vi "RunScript.vi"(6 "String Reference (Severity)":refnum<vi>, 7 "ScriptFileNames":path[](array[path]), 8 "Error In":errorcluster, 10 "File Path to Python Script":path, 11 "Python or INIScript?":T1=enum."Python") -> (0 "Error Out":errorcluster, 1 "Valid File Path":bool, 2 "File Path Control Out":path, 3 "Python Script Window":bool, 4 "INI Script Name Out":string)   [LabVIEW 2018]
doc: "This VI allows the which Script (Python or INI file) to run and/or whether to enable automatic error handling and leave the python script command window open to aid in debuging."
uses:
  TypeDefs/PythonOrINIScript.ctl
  NistPluggableModules/TestClass/Test.lvclass
panel:
  in  "INI Script Name":u16(ring) items=["*AbortScript", "*Start", "*Stop", "*AutoTimeout", "*Script", "*T", "*TT0", "*TT1"]
  in  "Cancel Button":bool
  in  "Auto In":bool
  in  "Done Button":bool
  in  "PSW In":bool
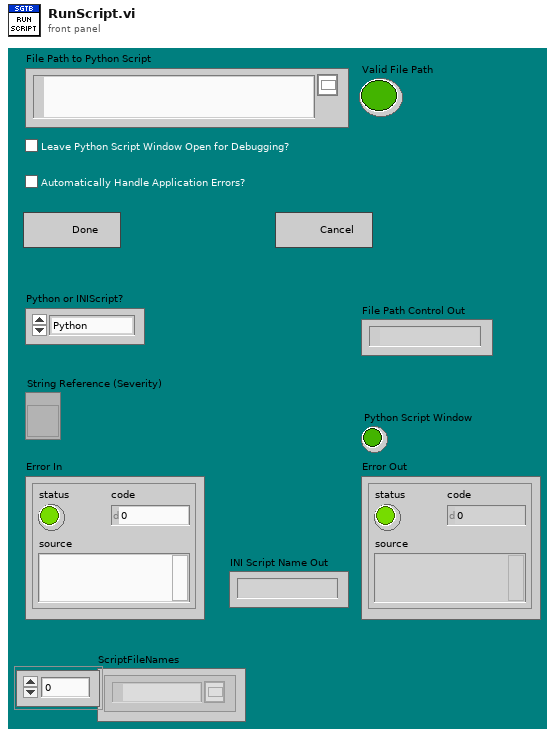
[diagram p1: front panel]
types:
  T1 = typedef "PythonOrINIScript.ctl" = enum16{"INIScript", "Python"}
  T2 = enum32{"Invalid", "Standard", "Closed", "Hidden", "Minimized", "Maximized"}
  T3 = enum32{"Invalid", "Default", "Floating", "Floating/Auto-Hide", "Modal"}
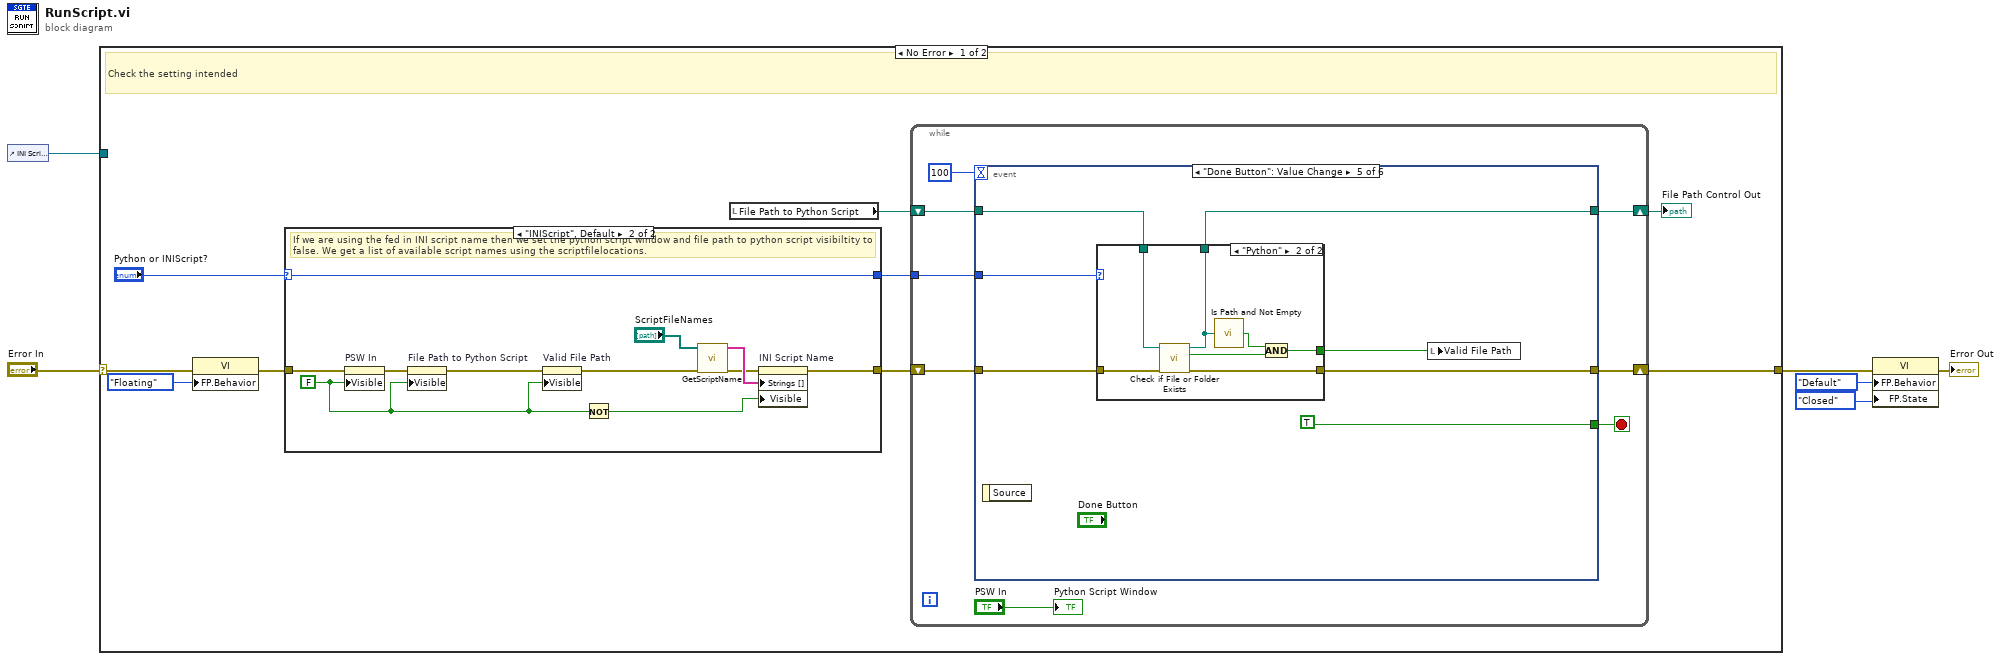
[diagram p0: block diagram]
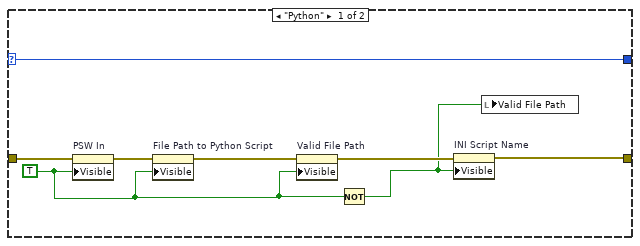
[diagram p2: hidden frame]
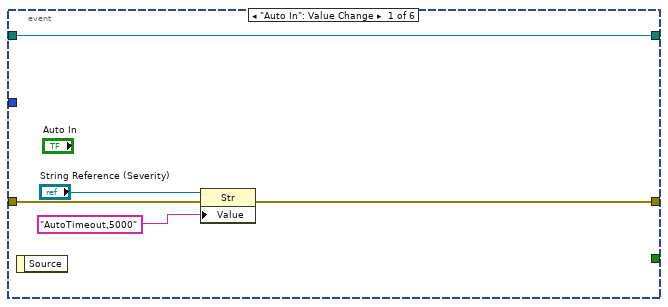
[diagram p3: hidden frame]
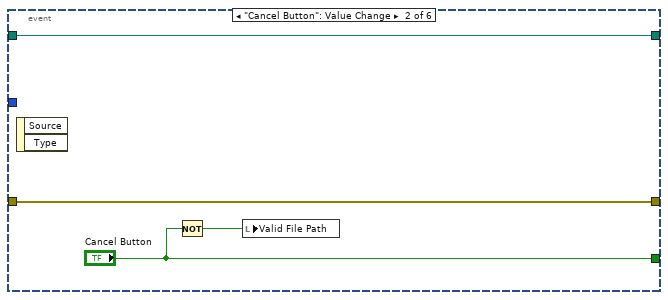
[diagram p4: hidden frame]
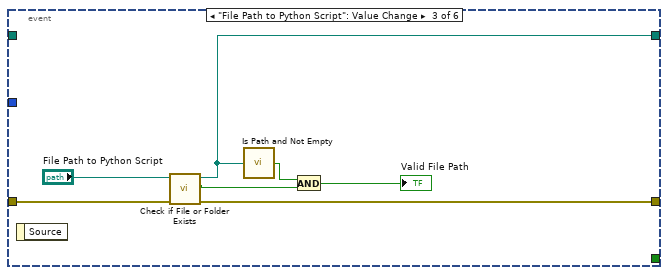
[diagram p5: hidden frame]
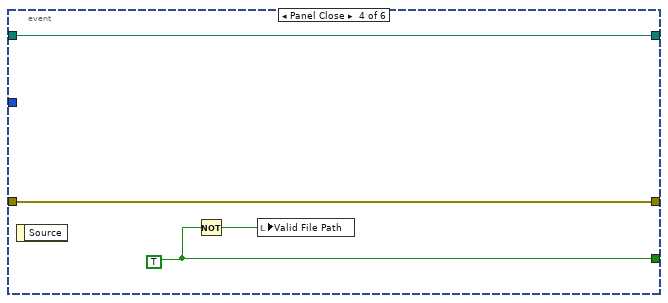
[diagram p6: hidden frame]
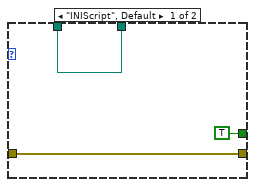
[diagram p7: hidden frame]
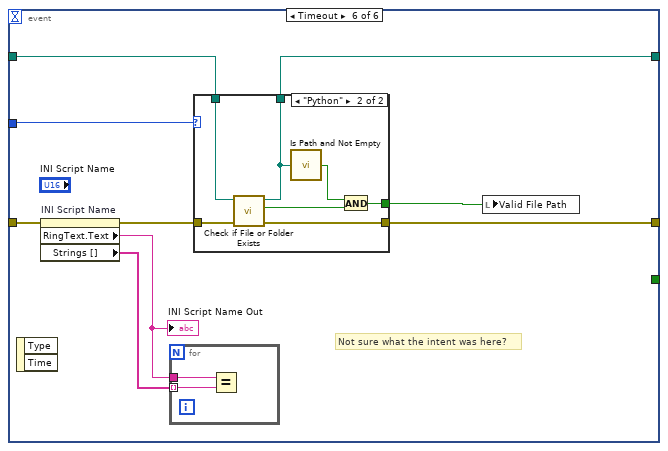
[diagram p8: hidden frame]
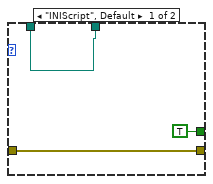
[diagram p9: hidden frame]
diagram:
  n1 = control-ref of="INI Script Name"() -> (w1:refnum<vi>)
  n2 = case shown="No Error" "Error In" {
    selector: "Error In" -> [w14 w101]
    tunnel: [w12 w101] -> w4
    tunnel: w1 -> [_ _]
    frame No Error {
      # "Check the setting intended"
      n3 = property class="VI"(error in=w14, "FP.Behavior"=T3."Floating" ("Front Panel Window:Behavior")) -> (error out=w13:errorcluster)  [unwired: 1 in, 1 out]
      n4 = case shown="\"INIScript\", Default" "Python or INIScript?" {
        selector: "Python or INIScript?" -> [w16 w24]
        tunnel: w13 -> [w23 w34]
        tunnel: [w19 w30] -> w11
        tunnel: [w16 w24] -> w7
        frame "Python" {
          w20 = TRUE ("Visible")
          n5 = property on="PSW In" class="Bool (strict)"(error in=w23, "Visible"=w20) -> (error out=w22:errorcluster)  [unwired: 1 in, 1 out]
          n6 = property on="File Path to Python Script" class="Path"(error in=w22, "Visible"=w20) -> (error out=w21:errorcluster)  [unwired: 1 in, 1 out]
          n7 = property on="Valid File Path" class="Bool (strict)"(error in=w21, "Visible"=w20) -> (error out=w18:errorcluster)  [unwired: 1 in, 1 out]
          n8 = Not(x=w20) -> (.not. x?=w17:bool)
          n9 = property on="INI Script Name" class="Ring (strict)"(error in=w18, "Visible"=w17) -> (error out=w19:errorcluster)  [unwired: 1 in, 1 out]
          n10 = local write "Valid File Path"(w17) -> ()
        }
        frame "INIScript", Default {
          w31 = FALSE ("Visible")
          # "If we are using the fed in INI script name then we set the python script window and file path to python script visibiltity to false. We get a list of available script names using the scriptfilelocations."
          n11 = property on="PSW In" class="Bool (strict)"(error in=w34, "Visible"=w31) -> (error out=w33:errorcluster)  [unwired: 1 in, 1 out]
          n12 = property on="File Path to Python Script" class="Path"(error in=w33, "Visible"=w31) -> (error out=w32:errorcluster)  [unwired: 1 in, 1 out]
          n13 = property on="Valid File Path" class="Bool (strict)"(error in=w32, "Visible"=w31) -> (error out=w27:errorcluster)  [unwired: 1 in, 1 out]
          n14 = Not(x=w31) -> (.not. x?=w29:bool)
          n15 = call "GetScriptName.vi"("error in"=w27, "ConfigINIFiles"="ScriptFileNames") -> ("error out"=w25:errorcluster, "Script Names"=w26:string[])  [unwired: 8 in]
          n16 = property on="INI Script Name" class="Ring (strict)"(error in=w25, "Strings []"=w26, "Visible"=w29) -> (error out=w30:errorcluster)  [unwired: 1 in, 1 out]
        }
      }
      n17 = local read "File Path to Python Script"() -> (w8:path)
      n18 = while {
        shift-right: [w42] -> w12
        shift-left: w11 -> [w41]
        shift-right: [w38] -> w10
        shift-left: w8 -> [w37]
        tunnel: w7 -> [w35]
        stop <- w40 stop-if-true
        n19 = event shown="[4] \"Done Button\": Value Change" {
          selector: _ -> [_ _ _ _ _ _]
          dyn-events: _ -> [_ _ _ _ _ _]
          timeout: 100 -> [_ _ _ _ _ _]
          tunnel: w41 -> [w47 w51 w58 w62 w67 w88]
          tunnel: [w43 w51 w57 w62 w66 w86] -> w42
          tunnel: [_ "Cancel Button" _ w60 TRUE ("Stop Button") _] -> w40
          tunnel: [w44 w50 w54 w61 w65 w84] -> w38
          tunnel: w37 -> [w44 w50 _ w61 w68 w85]
          tunnel: w35 -> [_ _ _ _ w63 w80]
          event "Auto In": Value Change {
            n20 = event-data() -> ()  [unwired: 1 in, 1 out]
            n21 = property class="Str"(reference="String Reference (Severity)", error in=w47, "Value"="AutoTimeout,5000" ("String")) -> (error out=w43:errorcluster)  [unwired: 1 out]
          }
          event "Cancel Button": Value Change {
            n22 = event-data() -> ()  [unwired: 1 in, 2 out]
            n23 = Not(x="Cancel Button") -> (.not. x?=w48:bool)
            n24 = local write "Valid File Path"(w48) -> ()
          }
          event "File Path to Python Script": Value Change {
            n25 = event-data() -> ()  [unwired: 1 in, 1 out]
            n26 = call <vilib>:"Check if File or Folder Exists.vi"("error in (no error)"=w58, "path"="File Path to Python Script") -> ("error out"=w57:errorcluster, "file or folder exists?"=w53:bool, "dup path"=w54:path)  [unwired: 7 in]
            n27 = call <vilib>:"Is Path and Not Empty.vi"("path"=w54) -> ("Is Path and Not Empty?"=w55:bool)  [unwired: 4 in]
            n28 = And(x=w55, y=w53) -> (x .and. y?=→"Valid File Path":bool)
          }
          event Panel Close {
            w60 = TRUE ("Stop Button")
            n29 = event-data() -> ()  [unwired: 1 in, 1 out]
            n30 = Not(x=w60) -> (.not. x?=w59:bool)
            n31 = local write "Valid File Path"(w59) -> ()
          }
          event "Done Button": Value Change {
            n32 = event-data() -> ()  [unwired: 1 in, 1 out]
            n33 = case shown="\"Python\"" w63 {
              tunnel: w68 -> [w71 w79]
              tunnel: w67 -> [w72 w78]
              tunnel: [w72 w77] -> w66
              tunnel: [w71 w75] -> w65
              tunnel: [TRUE w73] -> w64
              frame "INIScript", Default {
              }
              frame "Python" {
                n34 = call <vilib>:"Check if File or Folder Exists.vi"("error in (no error)"=w78, "path"=w79) -> ("error out"=w77:errorcluster, "file or folder exists?"=w74:bool, "dup path"=w75:path)  [unwired: 7 in]
                n35 = call <vilib>:"Is Path and Not Empty.vi"("path"=w75) -> ("Is Path and Not Empty?"=w76:bool)  [unwired: 4 in]
                n36 = And(x=w76, y=w74) -> (x .and. y?=w73:bool)
              }
            }
            n37 = local write "Valid File Path"(w64) -> ()
          }
          event Timeout {
            # "Not sure what the intent was here?"
            n38 = event-data() -> ()  [unwired: 1 in, 2 out]
            n39 = property on="INI Script Name" class="Ring (strict)"(error in=w88) -> (error out=w87:errorcluster, "RingText.Text"=w81:string, "Strings []"=w82:string[])  [unwired: 1 in, 1 out]
            "INI Script Name Out" <- w81
            n40 = for {
              tunnel: w82 -> [w100] mode=indexing
              tunnel: w81 -> [w99]
              n41 = Equal?(x=w99, y=w100) -> ()  [unwired: 1 out]
            }
            n42 = case shown="\"Python\"" w80 {
              tunnel: w87 -> [w91 w98]
              tunnel: [w91 w97] -> w86
              tunnel: w85 -> [w89 w96]
              tunnel: [w89 w94] -> w84
              tunnel: [TRUE w92] -> w83
              frame "INIScript", Default {
              }
              frame "Python" {
                n43 = call <vilib>:"Check if File or Folder Exists.vi"("error in (no error)"=w98, "path"=w96) -> ("error out"=w97:errorcluster, "file or folder exists?"=w93:bool, "dup path"=w94:path)  [unwired: 7 in]
                n44 = call <vilib>:"Is Path and Not Empty.vi"("path"=w94) -> ("Is Path and Not Empty?"=w95:bool)  [unwired: 4 in]
                n45 = And(x=w95, y=w93) -> (x .and. y?=w92:bool)
              }
            }
            n46 = local write "Valid File Path"(w83) -> ()
          }
        }
        "Python Script Window" <- "PSW In"
      }
      "File Path Control Out" <- w10
    }
    frame Error {
    }
  }
  n47 = property class="VI"(error in=w4, "FP.Behavior"=T3."Default" ("Front Panel Window:Behavior"), "FP.State"=T2."Closed" ("Front Panel Window:State")) -> (error out=→"Error Out":errorcluster)  [unwired: 1 in, 1 out]
